vi "Draw Glyph.vi"(5 "Transform (Center)":refnum<class "Transform.lvclass">, 6 "Colors":T1={"Front"={"Color"=0, "Alpha"=255}, "Back"={"Color"=16448250, "Alpha"=255}}, 7 "Font (System)":refnum<class "Font Settings.lvclass">, 8 "error in (no error)":errorcluster, 9 "Destination":refnum<class "Glyph Canvas.lvclass">, 10 "codepoint":u32, 11 "Drawer In":refnum<class "Freetype Drawer.lvclass">) -> (0 "error out":errorcluster, 1 "Destination Out":refnum<class "Glyph Canvas.lvclass">, 3 "Drawer Out":refnum<class "Freetype Drawer.lvclass">)   [LabVIEW 2023, in "Freetype Drawer.lvlib" / "Freetype Drawer.lvclass"]
uses:
  Freetype Drawer.lvclass
  Font Glyph Drawer Interface/Glyph Canvas/Glyph Canvas.lvclass
  Font Glyph Drawer Interface/Font Settings/Font Settings.lvclass
  Font Glyph Drawer Interface/Transform/Transform.lvclass
  Freetype Drawer.lvlib
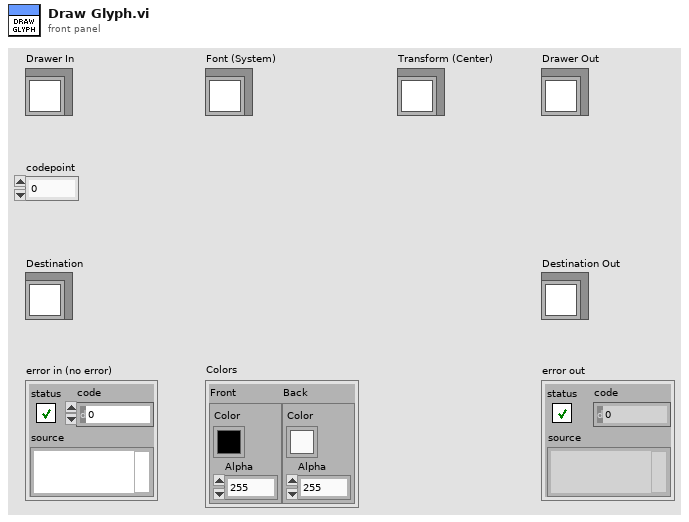
[diagram p1: front panel]
types:
  T1 = cluster{"Front":cluster{"Color":u32, "Alpha":u8}, "Back":cluster{"Color":u32, "Alpha":u8}}
  T2 = typedef "imagedata.ctl" = cluster{"image type":i32, "image depth":i32, "image":u8[], "mask":u8[], "colors":u32[], "Rectangle":cluster{"left":i16, "top":i16, "right":i16, "bottom":i16}}
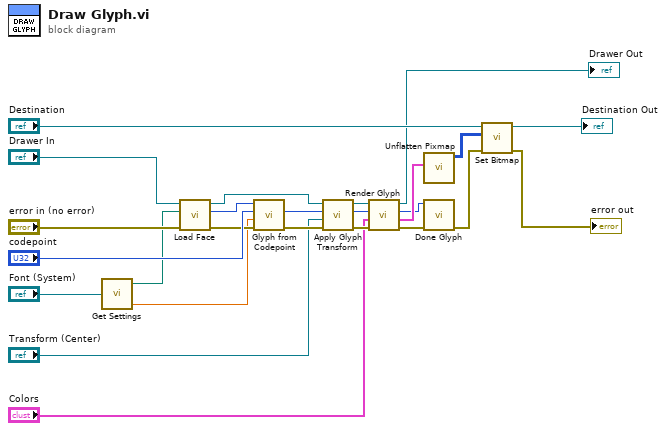
[diagram p0: block diagram]
diagram:
  n1 = call "Get Settings.vi"("Font Settings in"="Font (System)") -> ("Font Path"=w12:path, "Size"=w1:dbl)  [unwired: 1 out]
  n2 = call "Load Face.vi"("error in (no error)"="error in (no error)", "Font Path"=w12, "Freetype Drawer in"="Drawer In") -> ("error out"=w15:errorcluster, "face ref"=w14:i64, "Freetype Drawer out"=w10:refnum<class "Freetype Drawer.lvclass">)  [unwired: 6 in]
  n3 = call "Glyph from Codepoint.vi"("error in (no error)"=w15, "Size"=w1, "codepoint"="codepoint", "face ref"=w14) -> ("error out"=w18:errorcluster, "glyph ref out"=w9:i64)  [unwired: 5 in, 1 out]
  n4 = call "Apply Glyph Transform.vi"("error in (no error)"=w18, "Transform in"="Transform (Center)", "glyph ref in"=w9, "Drawer"=w10) -> ("error out"=w13:errorcluster, "glyph ref out"=w6:i64, "Drawer Out"=w7:refnum<class "Freetype Drawer.lvclass">)  [unwired: 5 in]
  n5 = call "Render Glyph.vi"("error in (no error)"=w13, "Colors"="Colors", "glyph ref in"=w6, "Freetype Drawer in"=w7) -> ("error out"=w17:errorcluster, "image data"=w4:T2, "glyph ref out"=w3:i64, "Freetype Drawer out"=→"Drawer Out":refnum<class "Freetype Drawer.lvclass">)  [unwired: 4 in]
  n6 = call <vilib>:"Unflatten Pixmap.vi"("image data"=w4) -> ("24-bit pixmap"=w23:u32[][])  [unwired: 4 in, 6 out]
  n7 = call "Done Glyph.vi"("error in (no error)"=w17, "glyph ref in"=w3) -> ("error out"=w22:errorcluster)  [unwired: 9 in]
  n8 = call-dynamic "Set Bitmap.vi"("error in (no error)"=w22, "Bitmap"=w23, "Glyph Canvas in"="Destination") -> ("error out"=→"error out":errorcluster, "Glyph Canvas out"=→"Destination Out":refnum<class "Glyph Canvas.lvclass">)  [unwired: 7 in]
